vi "Find out of Family.vi"(11 "filenames":string[](array[string])) -> (2 "Found":bool, 3 "Out of Family":string)   [LabVIEW 2023]
uses:
  <userlib>/_OpenG.lib/file/file.llb/Strip Path Extension - String__ogtk.vi
  <vilib>/Analysis/NI_AALBase.lvlib
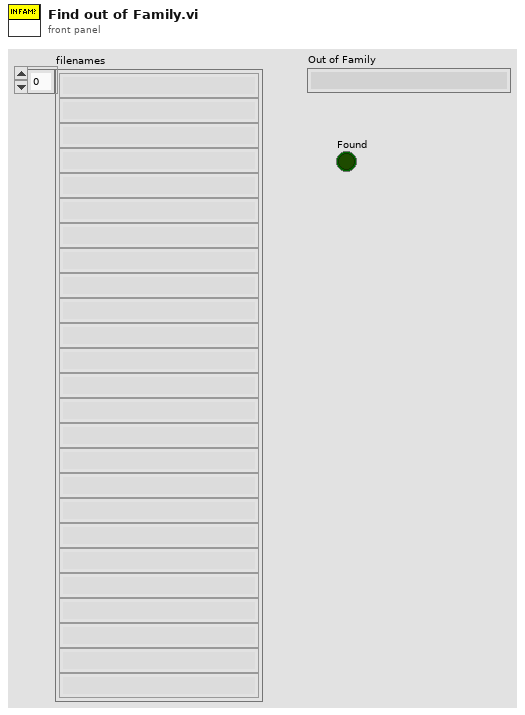
[diagram p1: front panel]
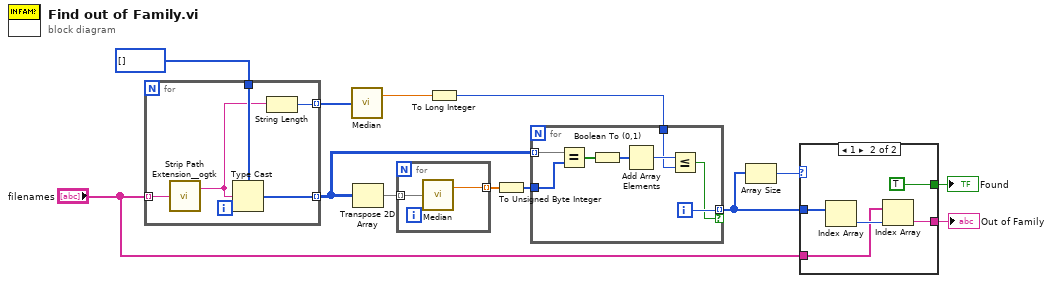
[diagram p0: block diagram]
diagram:
  n1 = for {
    tunnel: "filenames" -> [w15] mode=indexing
    tunnel: u8[] [] -> [w18]
    tunnel: [w17] -> w11 mode=indexing
    tunnel: [w16] -> w4 mode=indexing
    n2 = call-poly <userlib>:"Strip Path Extension__ogtk.vi"("path"=w15) -> ("root"=w14:string)  [unwired: 1 out]
    n3 = Type Cast(type=w18, x=w14) -> (*(type *) &x=w17:u8[])
    n4 = String Length(string=w14) -> (length=w16:i32)
  }
  n5 = call <vilib>:"Median.vi"("X"=w4) -> ("median"=w3:dbl)  [unwired: 1 out]
  n6 = Transpose 2D Array(2D array=w11) -> (transposed array=w12:u8[][])
  n7 = for {
    tunnel: w12 -> [w20] mode=indexing
    tunnel: [w19] -> w10 mode=indexing
    n8 = call <vilib>:"Median.vi"("X"=w20) -> ("median"=w19:dbl)  [unwired: 1 out]
  }
  n9 = To Long Integer(number=w3) -> (32bit integer=w2:i32)
  n10 = To Unsigned Byte Integer(number=w10) -> (unsigned 8bit integer=w9:u8[])
  n11 = for {
    tunnel: w11 -> [w28] mode=indexing
    tunnel: w9 -> [w27]
    tunnel: [w23] -> w7 mode=indexing if=w22
    tunnel: w2 -> [w21]
    i -> [w23]
    n12 = Equal?(x=w28, y=w27) -> (x = y?=w26:bool[])
    n13 = Boolean To (0,1)(Boolean=w26) -> (0, 1=w25:i16[])
    n14 = Add Array Elements(numeric array=w25) -> (sum=w24:i16)
    n15 = Less Or Equal?(x=w24, y=w21) -> (x <= y?=w22:bool)
  }
  n16 = Array Size(array=w7) -> (size(s)=w8:i32)
  n17 = case shown="1" w8 {
    tunnel: w7 -> [_ w33]
    tunnel: "filenames" -> [_ w31]
    tunnel: [_ w30] -> w6
    tunnel: [_ TRUE] -> w5
    frame Default {
    }
    frame 1 {
      n18 = Index Array(array=w33) -> (element=w32:i32)  [unwired: 1 in]
      n19 = Index Array(array=w31, index=w32) -> (element=w30:string)
    }
  }
  "Out of Family" <- w6
  "Found" <- w5
